vi "HEWH Generate Scan List.vi"(10 "Panel":enum16{"Panel 1", "Panel 2", "Panel 3"}(ring), 11 "Panel":T1[][](array[typedef])) -> (1 "Panel List":string[](array[string]), 2 "Channel Number":string[](array[string]), 3 "Channel Label":string[](array[string]), 5 "MW100 Channel Label":string[](array[string]))   [LabVIEW 2019]
uses:
  Type Definitions/HEWH Channel Label.ctl
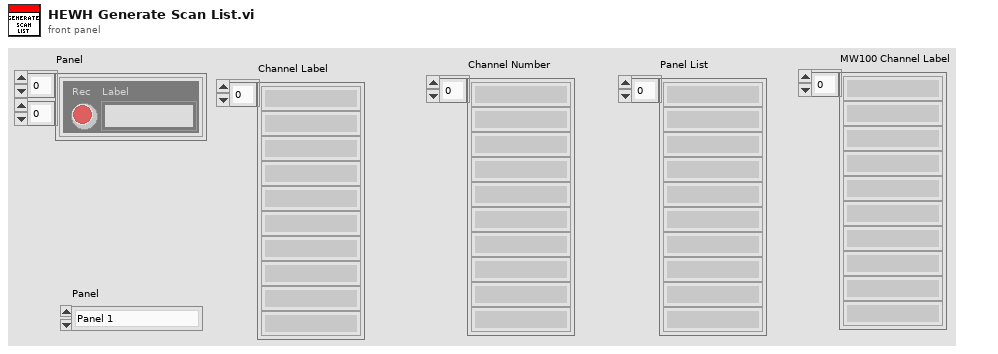
[diagram p1: front panel]
types:
  T1 = typedef "HEWH Channel Label.ctl" = cluster{"Label":string, "Chan":string, "Rec":bool}
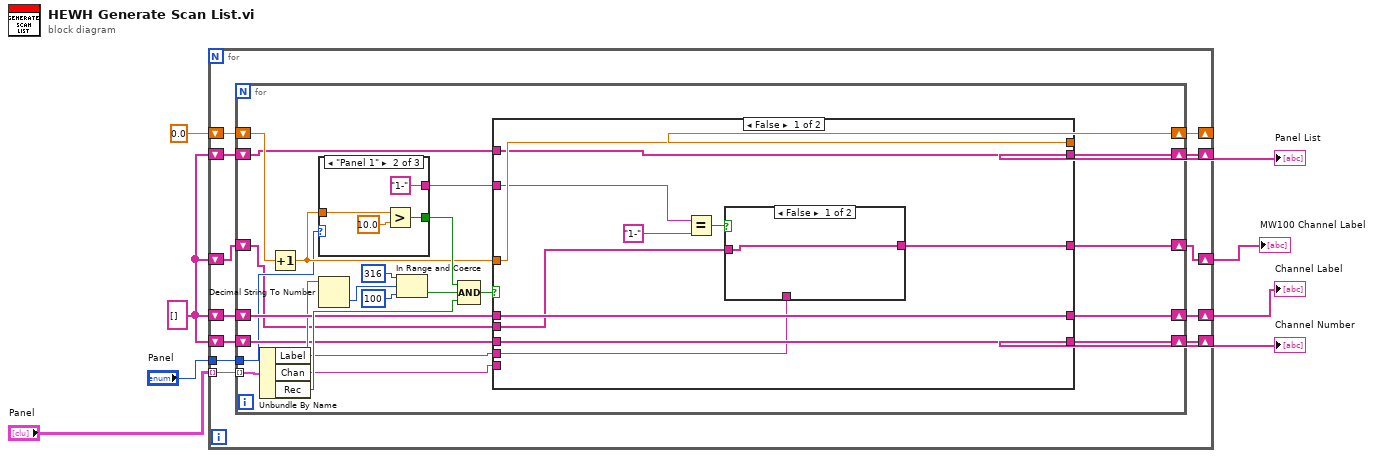
[diagram p0: block diagram]
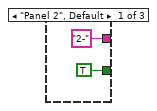
[diagram p2: hidden frame]
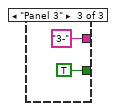
[diagram p3: hidden frame]
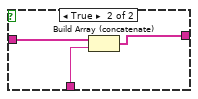
[diagram p4: hidden frame]
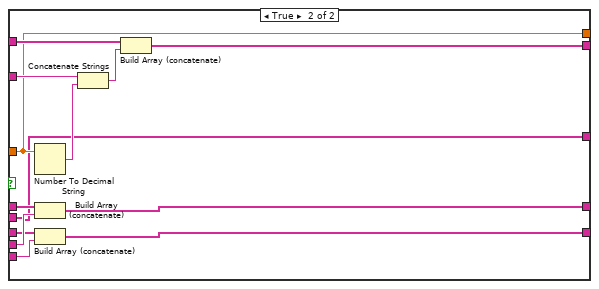
[diagram p5: hidden frame]
diagram:
  w1 = string[] []
  n1 = for {
    tunnel: "Panel" -> [w20] mode=indexing
    shift-right: [w19] -> w4
    shift-left: w1 -> [w18]
    shift-right: [w17] -> w3
    shift-left: w1 -> [w16]
    shift-right: [w14] -> _
    shift-left: 0.0 -> [w15]
    shift-right: [w12] -> w5
    shift-left: w1 -> [w13]
    tunnel: "Panel" -> [w11]
    shift-right: [w10] -> w2
    shift-left: w1 -> [w9]
    n2 = for {
      tunnel: w20 -> [w43] mode=indexing
      shift-right: [w35] -> w19
      shift-left: w18 -> [w29]
      shift-right: [w25] -> w17
      shift-left: w16 -> [w26]
      shift-right: [w34] -> w14
      shift-left: w15 -> [w37]
      shift-right: [w31] -> w12
      shift-left: w13 -> [w32]
      tunnel: w11 -> [w24]
      shift-right: [w22] -> w10
      shift-left: w9 -> [w21]
      n3 = Unbundle By Name(w43) -> ("Label"=w28:string, "Chan"=w27:string, "Rec"=w38:bool)
      n4 = Increment(x=w37) -> (x+1=w33:dbl)
      n5 = case shown="\"Panel 1\"" w24 {
        tunnel: [TRUE w48 TRUE] -> w36
        tunnel: w33 -> [_ w47 _]
        tunnel: ["2-" "1-" "3-"] -> w23
        frame "Panel 2", Default {
        }
        frame "Panel 1" {
          n6 = Greater?(x=w47, y=10.0) -> (0:w48:bool)
        }
        frame "Panel 3" {
        }
      }
      n7 = Decimal String To Number(string=w27) -> (number=w42:i32)  [unwired: 2 in, 1 out]
      n8 = In Range and Coerce(upper limit=316, x=w42, lower limit=100) -> (In Range?=w39:bool)  [unwired: 1 out]
      n9 = Compound Arithmetic op=AND(w36, w39, w38) -> (w30:bool)
      n10 = case shown="False" w30 {
        tunnel: w28 -> [w55 w78]
        tunnel: [w61 w77] -> w35
        tunnel: w29 -> [w61 w75]
        tunnel: [w58 w76] -> w25
        tunnel: w27 -> [_ w74]
        tunnel: w26 -> [w58 w73]
        tunnel: w33 -> [w60 w67]
        tunnel: [w59 w72] -> w31
        tunnel: [w60 w67] -> w34
        tunnel: w23 -> [w52 w71]
        tunnel: w32 -> [w59 w68]
        tunnel: [w57 w66] -> w22
        tunnel: w21 -> [w56 w66]
        frame False {
          n11 = Equal?(x=w52, y="1-") -> (x = y?=w54:bool)
          n12 = case shown="False" w54 {
            tunnel: [w62 w65] -> w57
            tunnel: w56 -> [w62 w64]
            tunnel: w55 -> [_ w63]
            frame False {
            }
            frame True {
              n13 = Build Array (concatenate)(w64, w63) -> (w65:string[])
            }
          }
        }
        frame True {
          n14 = Number To Decimal String(number=w67) -> (decimal integer string=w70:string)  [unwired: 1 in]
          n15 = Build Array (concatenate)(w75, w78) -> (w77:string[])
          n16 = Build Array (concatenate)(w73, w74) -> (w76:string[])
          n17 = Concatenate Strings(w71, w70) -> (w69:string)
          n18 = Build Array (concatenate)(w68, w69) -> (w72:string[])
        }
      }
    }
  }
  "Panel List" <- w5
  "Channel Number" <- w3
  "Channel Label" <- w4
  "MW100 Channel Label" <- w2
